vi "setControlTemperature.vi"(8 "error in (no error)":errorcluster, 10 "temperature in":sgl, 11 "CoolerControler in":refnum<class "CoolerControler.lvclass">) -> (0 "error out":errorcluster, 2 "temperature out":sgl, 3 "CoolerControler out":refnum<class "CoolerControler.lvclass">)   [LabVIEW 2016, in "CoolerControler.lvclass"]
uses:
  CoolerControler.lvclass
  typedefs/CoolerId.ctl
  SerialCommand/CoolerSerialCommand.lvclass
  typedefs/dataUnit.ctl
  typedefs/CoolerCommands.ctl
  CoolerControler.lvclass/CoolerControler.ctl
panel:
  in  "id":T1=1
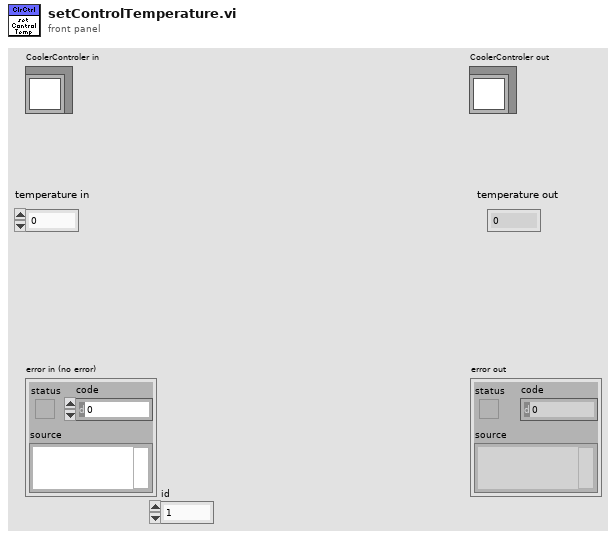
[diagram p1: front panel]
types:
  T1 = typedef "CoolerId.ctl" = u16
  T2 = typedef "CoolerCommands.ctl" = enum16{"None", "SetExternSensorStatus", "SetChillerStatus", "SetControlSensor", "SetControlTemperature", "SetHighSupplyTempWarning", "SetLowSupplyTemperatureWarning", "SetHighAmbientTemperatureWarning", "SetLowAmbienTemperatureWarning", "SetLowProcessFlowWarning", "SetHighSupplyTemperatureAlarm", "SetLowSupplyTemperatureAlarm", "SetHighAmbientTemperatureAlarm", "SetLowAmbientTemperatureAlarm", "SetLowProcessFlowAlarm"}
  T3 = typedef "dataUnit.ctl" = enum16{"temperature", "flow", "current", "PID", "fanSpeed", "time", "PWM", "TEDriveLevel", "Number"}
  T4 = typedef "response.ctl" = cluster{"deviceId":string, "commandNumber":string, "errorActive":bool, "commandName":string, "responseData":string, "checkSum":string}
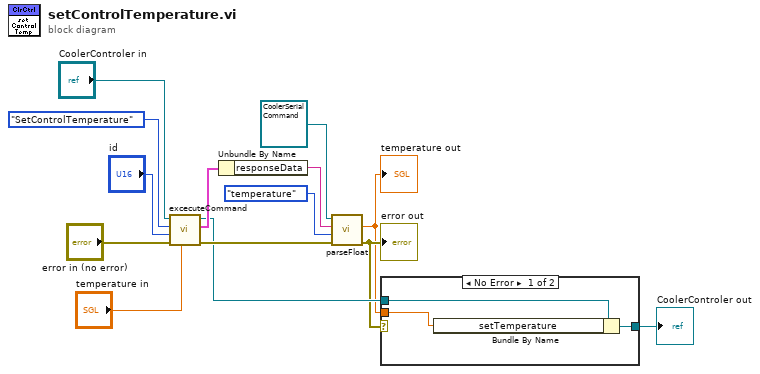
[diagram p0: block diagram]
diagram:
  n1 = call "excecuteCommand.vi"("inputValue"="temperature in", "error in (no error)"="error in (no error)", "id"="id", "CoolerCommand"=CoolerCommands."SetControlTemperature", "CoolerControler in"="CoolerControler in") -> ("error out"=w11:errorcluster, "response out"=w12:T4, "CoolerControler out"=w4:refnum<class "CoolerControler.lvclass">)  [unwired: 4 in]
  n2 = Unbundle By Name(w12) -> ("responseData"=w14:string)
  n3 = call "parseFloat.vi"("error in (no error)"=w11, "unit"=dataUnit."temperature", "commandData"=w14, "CoolerSerialCommand in"=refnum<class "CoolerSerialCommand.lvclass"> refnum) -> ("error out"=w3:errorcluster, "value"=w1:sgl)  [unwired: 4 in, 2 out]
  "error out" <- w3
  "temperature out" <- w1
  n4 = case shown="No Error" w3 {
    tunnel: w4 -> [w17 w18]
    tunnel: [w15 w18] -> w2
    tunnel: w1 -> [w16 _]
    frame No Error {
      n5 = Bundle By Name(cluster=w17, "setTemperature"=w16) -> (w15:refnum<class "CoolerControler.lvclass">)
    }
    frame Error {
    }
  }
  "CoolerControler out" <- w2
